vi "Stop Driving.vi"(7 "Description":string, 8 "Command Info In":T1) -> (0 "Command Info Out":T1)   [LabVIEW 2019]
doc: "Zero the drive motors, making the robot stationary."
uses:
  Implementation/Drive Operations.ctl
  Implementation/Drive Setpoints.ctl
  <vilib>/picture/picture.llb/imagedata.ctl
  Bordeaux/Command Stuff/Single Cmd Info.ctl
  <vilib>/Rock Robotics/WPI/Framework/Completion Status.ctl
  <vilib>/Rock Robotics/WPI/Framework/Completion Notifier.ctl
  <vilib>/Rock Robotics/WPI/Framework/Command Status Info.ctl
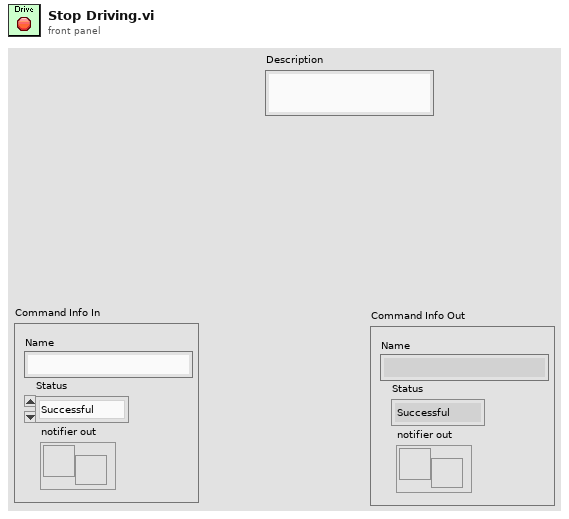
[diagram p1: front panel]
types:
  T1 = typedef "Command Status Info.ctl" = cluster{"Name":string, "Status":T2, "notifier out":T3}
  T2 = typedef "Completion Status.ctl" = enum16{"Successful", "Aborted", "Incomplete"}
  T3 = typedef "Completion Notifier.ctl" = refnum<notifier>
  T4 = typedef "Drive Setpoints.ctl" = cluster{"Operation":T5, "Forwards/Backwards":dbl, "Turning":dbl, "Transmition Engaged?":bool, "Reverse (T) / Normal (F)":bool, "Field Align?":bool, "Auto Path Data":cluster{"V":dbl[], "Theta":dbl[], "Sample Period":dbl}, "Path Reversed":bool, "Commands":cluster{"Time (s)":dbl, T6, bool}[]}
  T5 = typedef "Drive Operations.ctl" = enum16{"Reserve", "Read Current", "Immediate", "Pod Racer", "Ball AA", "Play Back From Log"}
  T6 = typedef "Single Cmd Info.ctl" = cluster{"Name":string, "CPTM.DataType":variant, "All Control Values Variant":cluster{"Name":string, "Variant Data":variant}[], "icon full":T7, "icon scaled":T7, "Path":path, "Subsystem Color":u32}
  T7 = typedef "imagedata.ctl" = cluster{"image type":i32, "image depth":i32, "image":u8[], "mask":u8[], "colors":u32[], "Rectangle":cluster{"left":i16, "top":i16, "right":i16, "bottom":i16}}
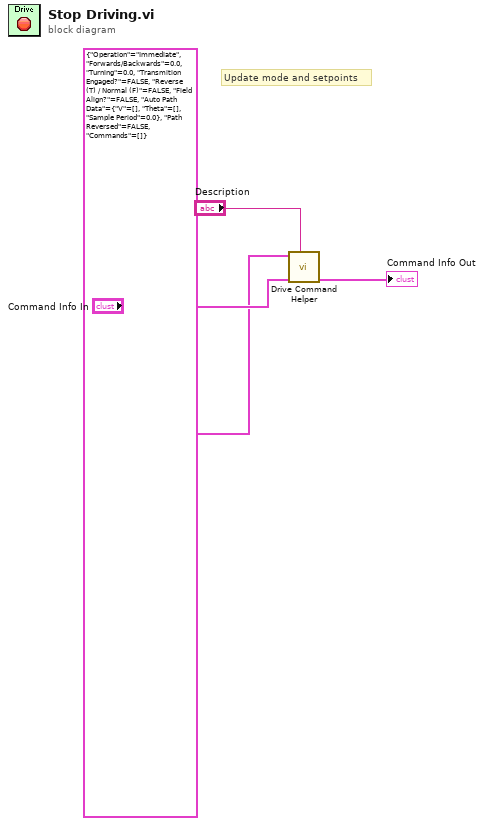
[diagram p0: block diagram]
diagram:
  # "Update mode and setpoints"
  n1 = call "Drive Command Helper.vi"("Description"="Description", "Command Info In"="Command Info In", "SubSystem Data"=T4 {"Operation"=enum."Immediate", "Forwards/Backwards"=0.0, "Turning"=0.0, "Transmition Engaged?"=FALSE, "Reverse (T) / Normal (F)"=FALSE, "Field Align?"=FALSE, "Auto Path Data"={"V"=[], "Theta"=[], "Sample Period"=0.0}, "Path Reversed"=FALSE, "Commands"=[]}) -> ("Command Info Out"=→"Command Info Out":T1)  [unwired: 6 in, 2 out]
